vi "niScope Configure Vertical.vi"(0 "instrument handle":refnum<k15>, 1 "probe attenuation":dbl=1.0 format="%.1f", 2 "vertical coupling":T1=1 items=["AC", "DC", "Ground"], 5 "channels":string="0", 7 "vertical range":dbl=10.0 format="%.2f", 9 "vertical offset":dbl format="%.4f", 11 "error in":errorcluster, 12 "channel enabled":bool=TRUE) -> (4 "instrument handle out":refnum<k15>, 15 "error out":errorcluster)   [LabVIEW 2013]
doc: "Configures the most commonly configured properties of the digitizer vertical subsystem, such as the range, offset, coupling, probe attenuation, and the channel name."
uses:
  <instrlib>/niScope/Controls/niScope vertical coupling.ctl
  niScope_32.dll
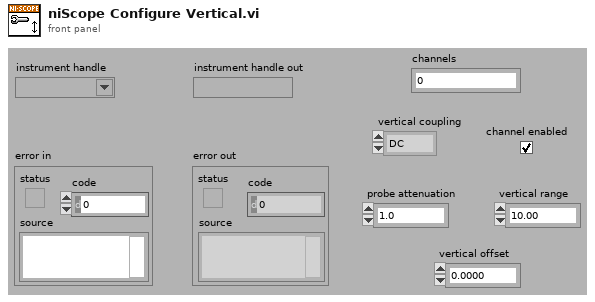
[diagram p1: front panel]
types:
  T1 = typedef "niScope vertical coupling.ctl" = i32
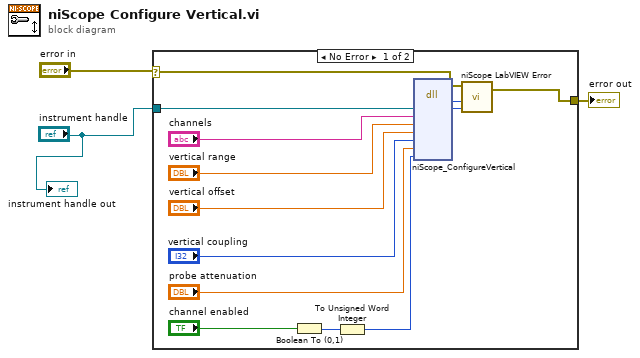
[diagram p0: block diagram]
diagram:
  n1 = case shown="No Error" "error in" {
    selector: "error in" -> [w4 w17]
    tunnel: [w6 w17] -> w2
    tunnel: "instrument handle" -> [w16 _]
    frame No Error {
      n2 = Boolean To (0,1)(Boolean="channel enabled") -> (0, 1=w10:i16)
      n3 = To Unsigned Word Integer(number=w10) -> (unsigned 16bit integer=w9:u16)
      n4 = dll-call lib="niScope_*.*" fn="niScope_ConfigureVertical"("instrument handle"=w16, "channel"="channels", "range"="vertical range", "offset"="vertical offset", "coupling"="vertical coupling", "probeAttenuation"="probe attenuation", "enabled"=w9) -> ("status"=w8:i32, "instrument handle"=w7:u32)  [unwired: 9 in, 2 out]
      n5 = call <instrlib>:"niScope LabVIEW Error.vi"("instrument handle"=w7, "niScope error code (0)"=w8, "error in (no error)"=w4) -> ("error out"=w6:errorcluster)  [unwired: 2 in]
    }
    frame Error {
    }
  }
  "error out" <- w2
  "instrument handle out" <- "instrument handle"
